vi "Agilent Read 5 Units.vi"(0 "Agilent Refs":refnum<visa-resource-name>[](array[refnum])=["AGILENT1", "AGILENT2", "AGILENT3", "AGILENT4", "AGILENT6"], 5 "error in (no error)":errorcluster, 6 "file path (dialog if empty)":path=path "C:/NI-2010/Trunk/Dryer Wilt/Agilent Channel Assignment - Wilt.ini", 10 "Agilent":T1) -> (14 "All Agilent Data":dbl[](array[numeric]), 19 "error out":errorcluster)   [LabVIEW 2012]
panel:
  in  "Tab Control":enum32{"Current Data", "Debug Data"}(tab)
  out "Array":T2(array[cluster])
  out "Num Agilent Data":i32
  out "Index Array":i32[][](array[numeric])
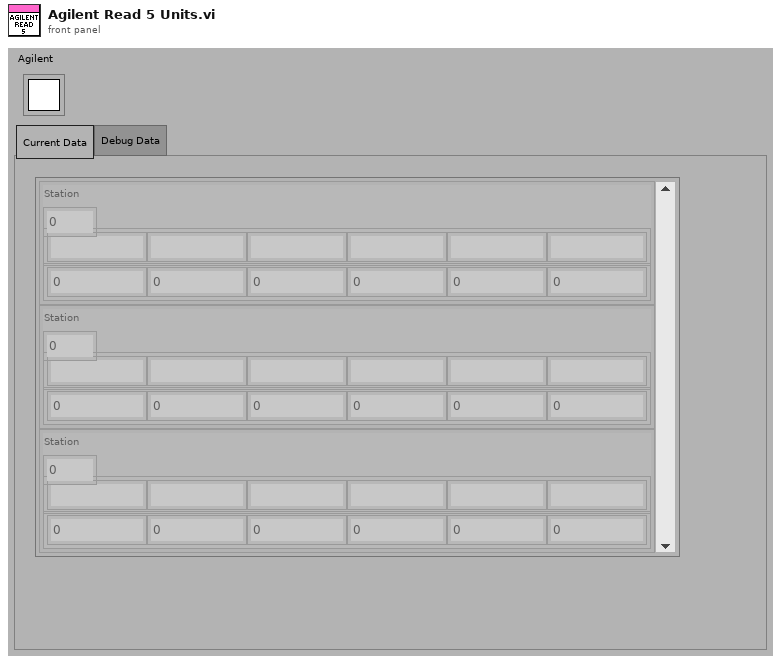
[diagram p1: front panel]
types:
  T1 = typedef "Semaphore RefNum" = refnum<k1>
  T2 = cluster{"Station":i32, "Station Data Headers":string[], dbl[]}[]
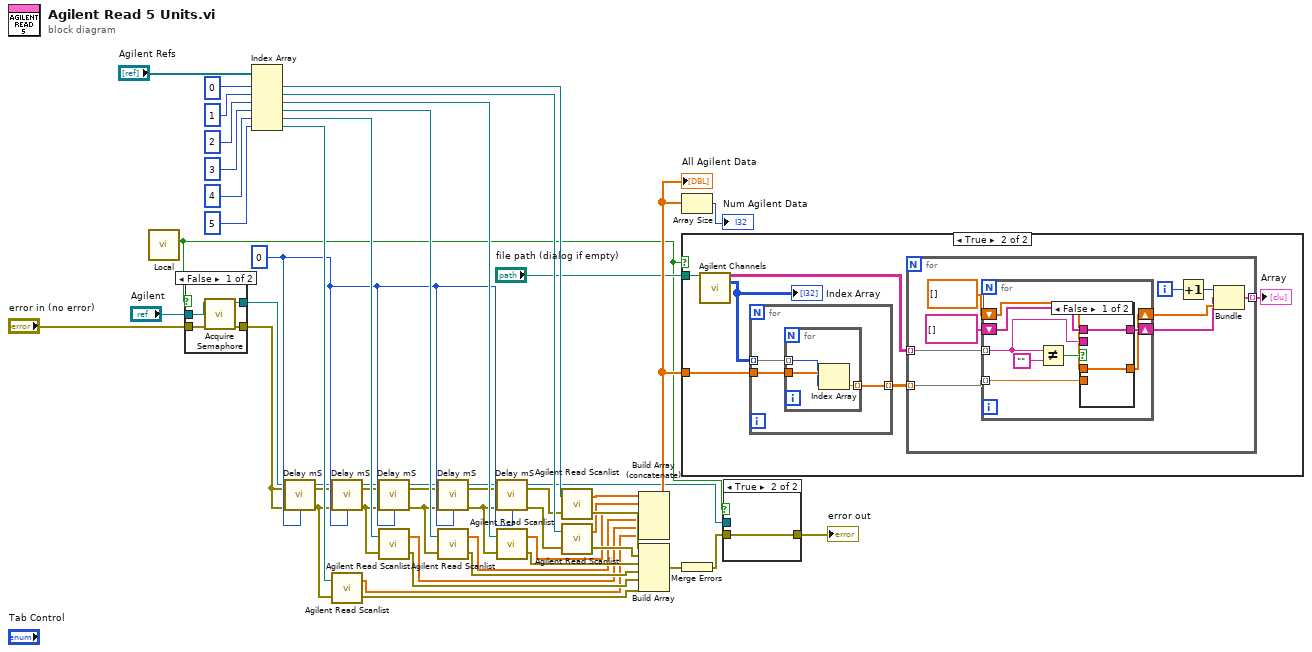
[diagram p0: block diagram]
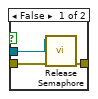
[diagram p2: hidden frame]
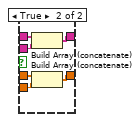
[diagram p5: hidden frame]
diagram:
  w13 = u32 0 ("milliseconds to wait")
  n1 = call "Local.vi"() -> ("Local?"=w1:bool)  [unwired: 11 in]
  n2 = case shown="False" w1 {
    tunnel: "error in (no error)" -> [w46 w48]
    tunnel: [w45 w48] -> w5
    tunnel: [w44 w47] -> w3
    tunnel: "Agilent" -> [w43 w47]
    frame False {
      n3 = call <vilib>:"Acquire Semaphore.vi"("error in (no error)"=w46, "semaphore"=w43) -> ("error out"=w45:errorcluster, "semaphore out"=w44:T1)  [unwired: 3 in, 1 out]
    }
    frame True {
    }
  }
  n4 = Index Array(array="Agilent Refs", index #1=0 ("index"), index #2=1 ("index"), index #3=2 ("index"), index #4=3 ("index"), index #5=4 ("index"), index #6=5 ("index")) -> (element #1=w36:refnum<visa-resource-name>, element #2=w30:refnum<visa-resource-name>, element #3=w25:refnum<visa-resource-name>, element #4=w24:refnum<visa-resource-name>, element #5=w21:refnum<visa-resource-name>, element #6=w16:refnum<visa-resource-name>)
  n5 = call "Delay mS.vi"("Error In"=w5, "milliseconds to wait"=w13) -> ("Error Out"=w9:errorcluster)  [unwired: 13 in]
  n6 = call "Delay mS.vi"("Error In"=w9, "milliseconds to wait"=w13) -> ("Error Out"=w10:errorcluster)  [unwired: 13 in]
  n7 = call "Agilent Read Scanlist.vi"("error in (no error)"=w9, "VISA Resource Name"=w16) -> ("error out"=w18:errorcluster, "Output Data (Numbers Only)"=w17:dbl[])
  n8 = call "Delay mS.vi"("Error In"=w10, "milliseconds to wait"=w13) -> ("Error Out"=w11:errorcluster)  [unwired: 13 in]
  n9 = call "Agilent Read Scanlist.vi"("error in (no error)"=w10, "VISA Resource Name"=w21) -> ("error out"=w20:errorcluster, "Output Data (Numbers Only)"=w19:dbl[])
  n10 = call "Delay mS.vi"("Error In"=w11, "milliseconds to wait"=w13) -> ("Error Out"=w12:errorcluster)  [unwired: 13 in]
  n11 = call "Agilent Read Scanlist.vi"("error in (no error)"=w11, "VISA Resource Name"=w24) -> ("error out"=w22:errorcluster, "Output Data (Numbers Only)"=w23:dbl[])
  n12 = call "Delay mS.vi"("Error In"=w12, "milliseconds to wait"=w13) -> ("Error Out"=w14:errorcluster)  [unwired: 13 in]
  n13 = call "Agilent Read Scanlist.vi"("error in (no error)"=w12, "VISA Resource Name"=w25) -> ("error out"=w26:errorcluster, "Output Data (Numbers Only)"=w27:dbl[])
  n14 = call "Agilent Read Scanlist.vi"("error in (no error)"=w5, "VISA Resource Name"=w36) -> ("error out"=w34:errorcluster, "Output Data (Numbers Only)"=w35:dbl[])
  n15 = call "Agilent Read Scanlist.vi"("error in (no error)"=w14, "VISA Resource Name"=w30) -> ("error out"=w29:errorcluster, "Output Data (Numbers Only)"=w28:dbl[])
  n16 = Build Array (concatenate)(w35, w28, w27, w23, w19, w17) -> (w7:dbl[])
  "All Agilent Data" <- w7
  n17 = Build Array(w34, w29, w26, w22, w20, w18) -> (w33:errorcluster[])
  n18 = Array Size(array=w7) -> (size(s)=→"Num Agilent Data":i32)
  n19 = case shown="True" w1 {
    tunnel: w7 -> [_ w52]
    tunnel: "file path (dialog if empty)" -> [_ w49]
    frame False {
    }
    frame True {
      n20 = call "Agilent Channels.vi"("file path (dialog if empty)"=w49) -> ("Station Data Headers"=w54:string[][], "Index Array"=w53:i32[][])  [unwired: 8 in, 5 out]
      "Index Array" <- w53
      n21 = for {
        tunnel: w53 -> [w56] mode=indexing
        tunnel: w52 -> [w57]
        tunnel: [w55] -> w51 mode=indexing
        n22 = for {
          tunnel: w57 -> [w60]
          tunnel: w56 -> [w59] mode=indexing
          tunnel: [w58] -> w55 mode=indexing
          n23 = Index Array(array=w60, index=w59) -> (element=w58:dbl)
        }
      }
      n24 = for {
        tunnel: w54 -> [w66] mode=indexing
        tunnel: w51 -> [w63] mode=indexing
        tunnel: [w69] -> w50 mode=indexing
        i -> [w68]
        n25 = for {
          tunnel: w66 -> [w76] mode=indexing
          shift-right: [w75] -> w61
          shift-left: string[] [] -> [w74]
          tunnel: w63 -> [w72] mode=indexing
          shift-right: [w71] -> w62
          shift-left: dbl[] [] -> [w70]
          n26 = Not Equal?(x=w76, y="") -> (x != y?=w73:bool)
          n27 = case shown="False" w73 {
            tunnel: w76 -> [_ w83]
            tunnel: [w79 w85] -> w75
            tunnel: w74 -> [w79 w84]
            tunnel: w72 -> [_ w82]
            tunnel: [w78 w81] -> w71
            tunnel: w70 -> [w78 w80]
            frame False {
            }
            frame True {
              n28 = Build Array (concatenate)(w84, w83) -> (w85:string[])
              n29 = Build Array (concatenate)(w80, w82) -> (w81:dbl[])
            }
          }
        }
        n30 = Increment(x=w68) -> (x+1=w67:i32)
        n31 = Bundle(w67, w61, w62) -> (w69:cluster{i32, string[], dbl[]})  [unwired: 1 in]
      }
      "Array" <- w50
    }
  }
  n32 = Merge Errors(w33) -> (w32:errorcluster)
  n33 = case shown="True" w1 {
    tunnel: w32 -> [w88 w89]
    tunnel: [w87 w89] -> w4
    tunnel: w3 -> [w86 _]
    frame False {
      n34 = call <vilib>:"Release Semaphore.vi"("error in (no error)"=w88, "semaphore"=w86) -> ("error out"=w87:errorcluster)  [unwired: 4 in, 1 out]
    }
    frame True {
    }
  }
  "error out" <- w4
